vi "Fact using shift register s.vi"() -> ()   [LabVIEW 2018]
panel:
  out "Numeric":dbl
  in  "n":i32
  out "avg of sum(n)":dbl
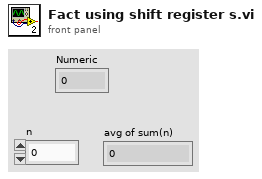
[diagram p1: front panel]
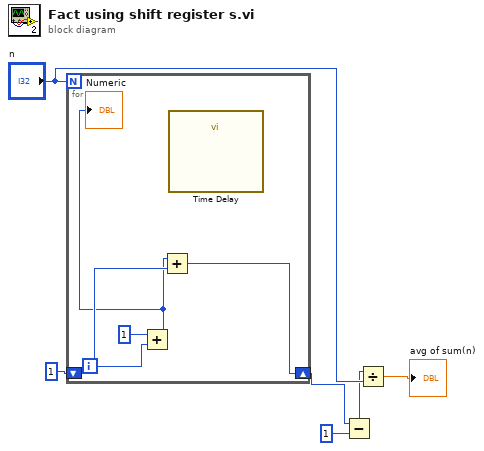
[diagram p0: block diagram]
diagram:
  n1 = for {
    N: "n" -> [_]
    shift-right: [w11] -> w3
    shift-left: 1 -> [w10]
    i -> [w8]
    n2 = Add(x=1, y=w8) -> (x+y=w7:i32)
    "Numeric" <- w7
    n3 = Add(x=w7, y=w10) -> (x+y=w11:i32)
    n4 = call "Time Delay"() -> ()  [unwired: 11 in, 1 out]
  }
  n5 = Subtract(x=w3, y=1) -> (x-y=w1:i32)
  n6 = Divide(x=w1, y="n") -> (x/y=→"avg of sum(n)":dbl)
